vi "SoftTrigger.vi"() -> ()   [LabVIEW 2017]
panel:
  in  "TriggerRate":u8(ring)=5 items=["125Hz", "250Hz", "500Hz", "1000Hz", "10000Hz", "20000Hz", "50000Hz"]
  in  "String":string
  in  "SoftTrigger":bool
  in  "address":string="192.168.10.35"
  in  "error in (no error)":errorcluster
  out "error out":errorcluster
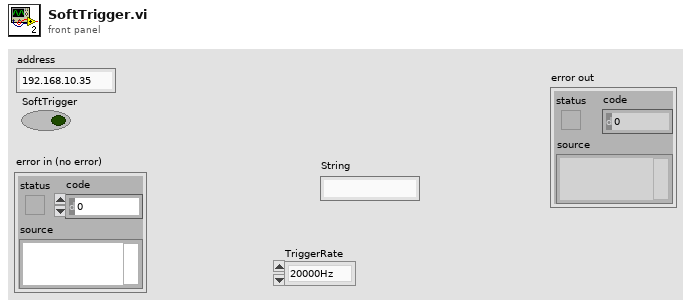
[diagram p1: front panel]
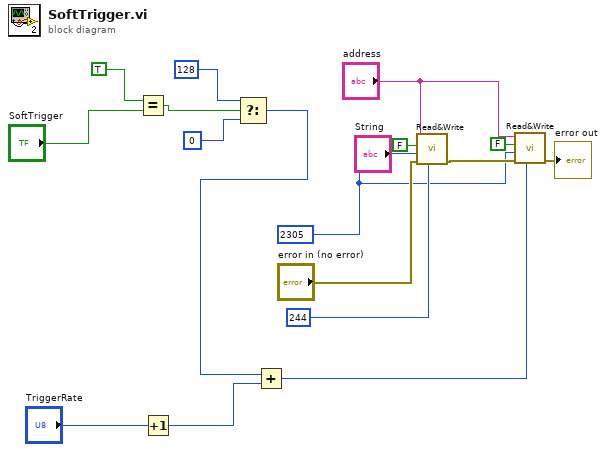
[diagram p0: block diagram]
diagram:
  w10 = u32 2305 ("Address")
  n1 = Equal?(x=TRUE, y="SoftTrigger") -> (x = y?=w8:bool)
  n2 = Increment(x="TriggerRate") -> (x+1=w3:u8)
  n3 = Select(t=u8 128 ("In 3"), s=w8, f=u8 0 ("In 3")) -> (s? t:f=w1:u8)
  n4 = Add(x=w1, y=w3) -> (x+y=w2:u8)
  n5 = call "Read&Write.vi"("In"=u8 244, "error in (no error)"="error in (no error)", "Address"=w10, "Read (TRUE)"=FALSE, "address"="address") -> ("error out"=w17:errorcluster)  [unwired: 5 in, 1 out]
  n6 = call "Read&Write.vi"("In"=w2, "error in (no error)"=w17, "Address"=w10, "Read (TRUE)"=FALSE, "address"="address") -> ("error out"=→"error out":errorcluster)  [unwired: 5 in, 1 out]
